vi "_refNumType.vi"(4 "Data":variant) -> (1 "Refnum Subtype Enum":T1(ring) format="%.0x")   [LabVIEW 2017, in "TagDB.lvlib"]
doc: "Gets the Refnum Type Enumeration of the input."
uses:
  TagDB.lvlib
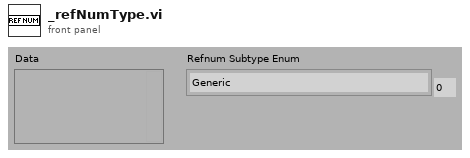
[diagram p1: front panel]
types:
  T1 = enum8{"Generic", "Datalog File Refnum", "Byte Stream File Refnum", "Device Refnum", "Occurence Refnum", "TCP Connection Refnum", "VISA Refnum (Obsolete)", "Automation Renum", "VI Server Refnum", "Menu Refnum", "IVI Refnum (Obsolete)", "IMAQ Session", "0x0C", "Datasocket Refnum", "VISA Resource", "IVI Logical Name", "UDP Connection Refnum", "Notifier Refnum", "Queue Refnum", "IrDA Refnum", "Hardware Plugin Refnum", "Hardware Plugin Tag Refnum", "DAQmx Refnum", "Event Registration Refnum", ".NET Refnum", "User Event Refnum", "0x1A", "Event Callback", "0x1C", "0x1D", "Only Used Internal to LabVIEW", "Bluetooth", "Data Value References", "RT FIFO", "TDM Streaming"}
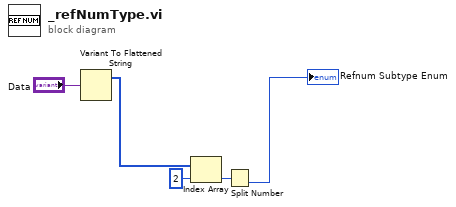
[diagram p0: block diagram]
diagram:
  n1 = Variant To Flattened String(Variant="Data") -> (1:w2:i16[])  [unwired: 1 out]
  n2 = Index Array(array=w2, index=2) -> (element=w3:i16)
  n3 = Split Number(x=w3) -> (lo(x)=→"Refnum Subtype Enum":u8)  [unwired: 1 out]
